vi "LakeShore Get Parameters.vi"(8 "error in (no error)":errorcluster, 10 "Control Panel Data":T1={"Record heater"=FALSE, "Record RAW"=FALSE, "Set point"=0.0, "Heater range"=0.0, "Approach"=enum."Instant", "Ramp rate, K/min"=0.0, "Record Channels"=[], "Settling time "=60.0, "Settling range"=0.1, "P"=0.0, "I"=0.0, "D"=0.0, "Temperature Control"=FALSE}, 11 "VISA resource name":refnum<visa-resource-name>) -> (0 "error out":errorcluster, 2 "Control Panel Data Out":T1={"Record heater"=FALSE, "Record RAW"=FALSE, "Set point"=0.0, "Heater range"=0.0, "Approach"=enum."Instant", "Ramp rate, K/min"=0.0, "Record Channels"=[], "Settling time "=60.0, "Settling range"=0.1, "P"=0.0, "I"=0.0, "D"=0.0, "Temperature Control"=FALSE}, 3 "VISA Resource Name Out":refnum<visa-resource-name>)   [LabVIEW 2015]
uses:
  Temperature Controller/Controls/T controller parameters.ctl
  Temperature Controller/Controls/Set Point Aproach.ctl
  GPIB/VISA  Send Receive.vi
panel:
  out "data string out":string
  out "data string":string
  # "Temperature Monitor"
  # "Temperature Monitor"
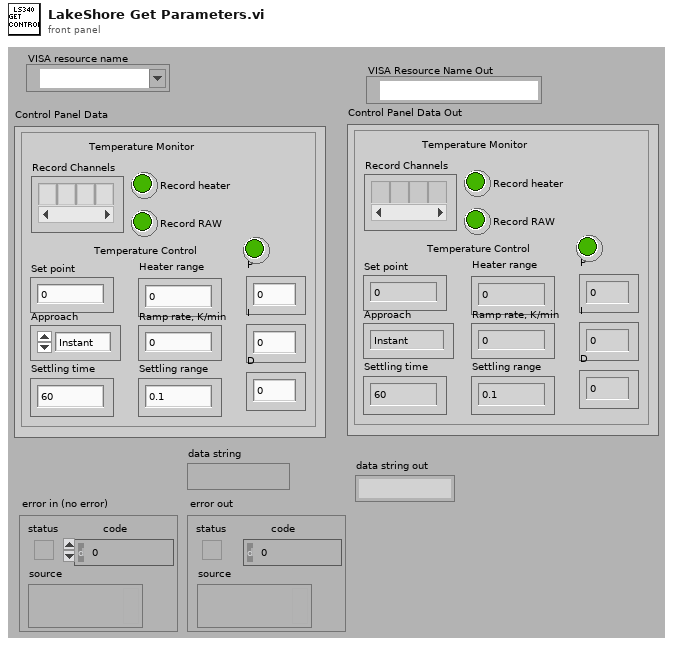
[diagram p1: front panel]
types:
  T1 = typedef "T controller parameters.ctl" = cluster{"Record heater":bool, "Record RAW":bool, "Set point":dbl, "Heater range":dbl, "Approach":T2, "Ramp rate, K/min":dbl, "Record Channels":string[], "Settling time ":dbl, "Settling range":dbl, "P":dbl, "I":dbl, "D":dbl, "Temperature Control":bool}
  T2 = typedef "Set Point Aproach.ctl" = enum16{"Instant", "Ramp"}
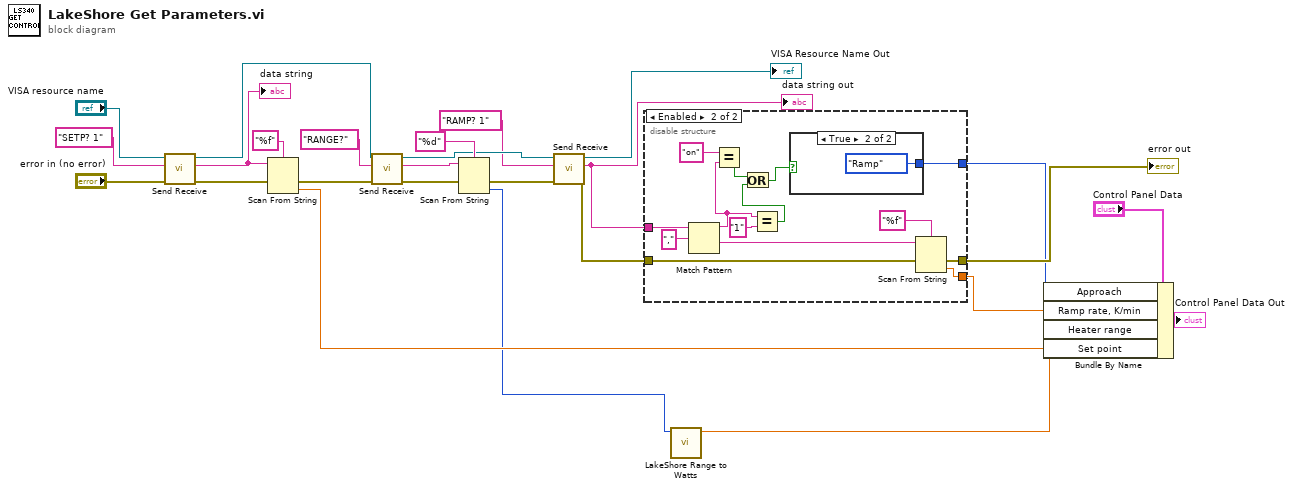
[diagram p0: block diagram]
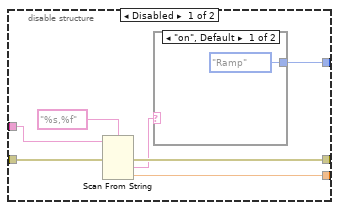
[diagram p2: hidden frame]
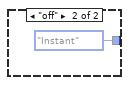
[diagram p3: hidden frame]
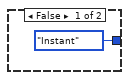
[diagram p4: hidden frame]
diagram:
  n1 = call-poly "Send Receive.vi"("error in (no error)"="error in (no error)", "data string in"="SETP? 1" ("data string"), "VISA Resource Name"="VISA resource name") -> ("error out"=w23:errorcluster, "data string out"=w19:string, "VISA Resource Name Out"=w12:refnum<visa-resource-name>)  [unwired: 6 in]
  "data string" <- w19
  n2 = Scan From String(format string="%f", input string=w19, error in=w23) -> (error out=w16:errorcluster, output 1=w4:dbl)  [unwired: 2 in, 2 out]
  n3 = call-poly "Send Receive.vi"("error in (no error)"=w16, "data string in"="RANGE?", "VISA Resource Name"=w12) -> ("error out"=w15:errorcluster, "data string out"=w14:string, "VISA Resource Name Out"=w13:refnum<visa-resource-name>)  [unwired: 6 in]
  n4 = Scan From String(format string="%d", input string=w14, error in=w15) -> (error out=w5:errorcluster, output 1=w2:i32)  [unwired: 2 in, 2 out]
  n5 = call-poly "Send Receive.vi"("error in (no error)"=w5, "data string in"="RAMP? 1" ("format string"), "VISA Resource Name"=w13) -> ("error out"=w18:errorcluster, "data string out"=w3:string, "VISA Resource Name Out"=→"VISA Resource Name Out":refnum<visa-resource-name>)  [unwired: 6 in]
  "data string out" <- w3
  n6 = disable-structure shown="Enabled" {
    disable-tunnel: w18 -> [w33 w45]
    disable-tunnel: [w32 w44] -> w11
    disable-tunnel: [w30 w49] -> w8
    disable-tunnel: [w29 w42] -> w7
    disable-tunnel: w3 -> [w28 w48]
    frame Disabled {
      n7 = Scan From String(format string="%s,%f", input string=w28, error in=w33) -> (error out=w32:errorcluster, output 1=w31:string, output 2=w29:dbl)  [unwired: 3 in, 2 out]
      n8 = case shown="\"on\", Default" w31 {
        tunnel: [Set_Point_Aproach."Ramp" ("Approach") Set_Point_Aproach."Instant" ("Approach")] -> w30
        frame "on", Default {
        }
        frame "off" {
        }
      }
    }
    frame Enabled {
      n9 = Match Pattern(string=w48, regular expression=",") -> (before substring=w38:string, after substring=w43:string)  [unwired: 1 in, 2 out]
      n10 = Equal?(x="on", y=w38) -> (x = y?=w36:bool)
      n11 = Equal?(x=w38, y="1" ("x")) -> (x = y?=w40:bool)
      n12 = Or(x=w36, y=w40) -> (x .or. y?=w39:bool)
      n13 = case shown="True" w39 {
        tunnel: [Set_Point_Aproach."Instant" ("Approach") Set_Point_Aproach."Ramp" ("Approach")] -> w49
        frame False {
        }
        frame True {
        }
      }
      n14 = Scan From String(format string="%f", input string=w43, error in=w45) -> (error out=w44:errorcluster, output 1=w42:dbl)  [unwired: 2 in, 2 out]
    }
  }
  "error out" <- w11
  n15 = call "LakeShore Range to Watts.vi"("Integer range"=w2) -> ("Watts"=w1:dbl)  [unwired: 9 in, 1 out]
  n16 = Bundle By Name(cluster="Control Panel Data", "Approach"=w8, "Ramp rate, K/min"=w7, "Heater range"=w1, "Set point"=w4) -> (→"Control Panel Data Out":T1)
